vi "Configure Voltage.vi"(0 "VISA resource name":refnum<visa-resource-name>, 1 "DB Reference (1)":dbl=1.0, 2 "Input Impedance (0: 10Mohm)":i32(ring) items=["10Mohm", "Auto"], 5 "Function (0: Voltage DC)":i32(ring) items=["Voltage DC"=0, "Voltage AC"=1, "Digitize Voltage"=13], 9 "Channel List(\"\")":string, 11 "error in (no error)":errorcluster, 12 "Unit (0: Volt)":i32(ring) items=["Volt", "DB"]) -> (4 "VISA resource name out":refnum<visa-resource-name>, 15 "error out":errorcluster)   [LabVIEW 2024, in "Keithley DMM6500 DAQ6500 Series.lvlib"]
doc: "Configures voltage settings, including DB reference, input impedance and unit."
uses:
  Keithley DMM6500 DAQ6500 Series.lvlib
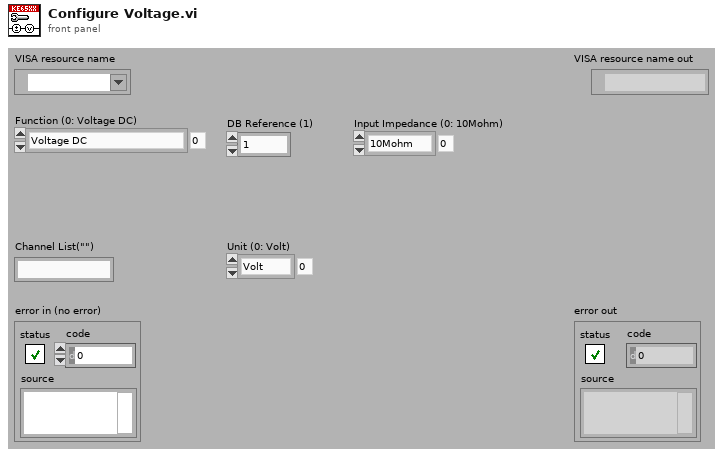
[diagram p1: front panel]
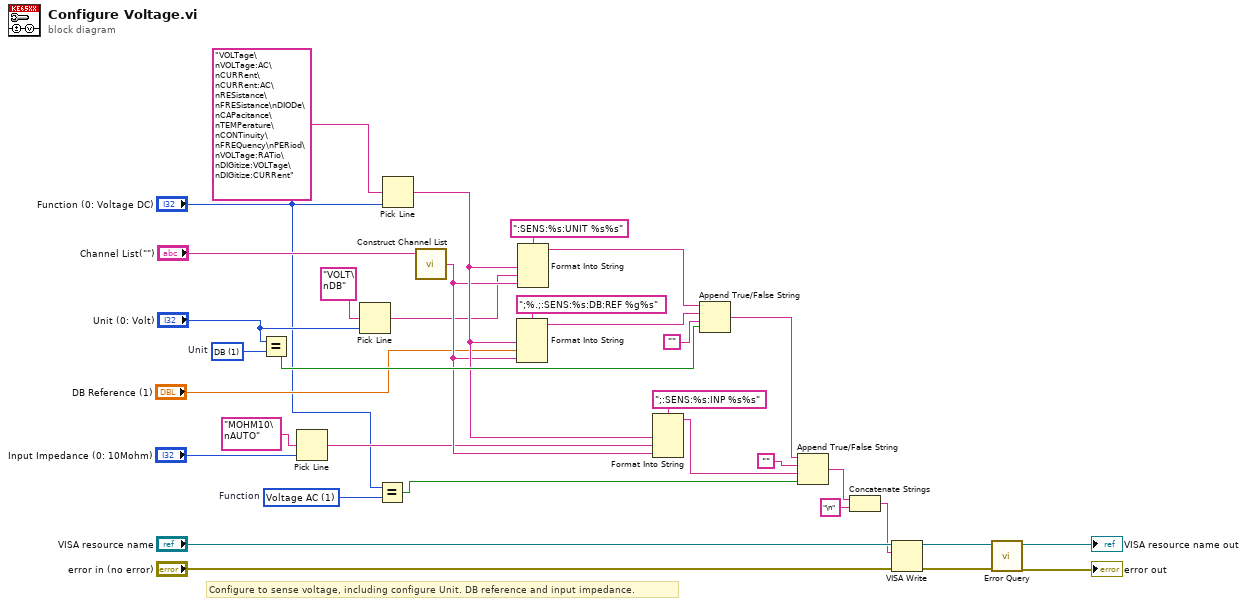
[diagram p0: block diagram]
diagram:
  w8 = u8 1 items=["Voltage DC"=0, "Voltage AC"=1, "Digitize Voltage"=13]  # Function
  w24 = u8 1 items=["VOLT", "DB"]  # Unit
  # "Configure to sense voltage, including configure Unit. DB reference and input impedance."
  n1 = Equal?(x="Unit (0: Volt)", y=w24) -> (x = y?=w22:bool)
  n2 = Pick Line(multi-line string="MOHM10\nAUTO", line index="Input Impedance (0: 10Mohm)") -> (output string=w10:string)  [unwired: 1 in]
  n3 = Pick Line(multi-line string="VOLT\nDB", line index="Unit (0: Volt)") -> (output string=w14:string)  [unwired: 1 in]
  n4 = Equal?(x="Function (0: Voltage DC)", y=w8) -> (x = y?=w7:bool)
  n5 = Pick Line(multi-line string="VOLTage\nVOLTage:AC\nCURRent\nCURRent:AC\nRESistance\nFRESistance\nDIODe\nCAPacitance\nTEMPerature\nCONTinuity\nFREQuency\nPERiod\nVOLTage:RATio\nDIGitize:VOLTage\nDIGitize:CURRent", line index="Function (0: Voltage DC)") -> (output string=w20:string)  [unwired: 1 in]
  n6 = call "Construct Channel List.vi"("Channel List"="Channel List(\"\")") -> ("Channel List String"=w19:string)  [unwired: 2 in]
  n7 = Format Into String(format string=";%.;:SENS:%s:DB:REF %g%s", w20, "DB Reference (1)", w19) -> (resulting string=w17:string)  [unwired: 2 in, 1 out]
  n8 = Format Into String(format string=":SENS:%s:UNIT %s%s", w20, w14, w19) -> (resulting string=w18:string)  [unwired: 2 in, 1 out]
  n9 = Format Into String(format string=";:SENS:%s:INP %s%s", w20, w10, w19) -> (resulting string=w6:string)  [unwired: 2 in, 1 out]
  n10 = Append True/False String(1:w22, 2:"" ("false string"), 3:w17, 4:w18) -> (0:w5:string)
  n11 = Append True/False String(1:w7, 2:w6, 3:"", 4:w5) -> (0:w2:string)
  n12 = Concatenate Strings(w2, "\n" ("string")) -> (w3:string)
  n13 = VISA Write(VISA resource name="VISA resource name", write buffer=w3, error in (no error)="error in (no error)") -> (VISA resource name out=w29:refnum<visa-resource-name>, error out=w28:errorcluster)  [unwired: 1 out]
  n14 = call "Error Query.vi"("error in (no error)"=w28, "VISA resource name"=w29) -> ("error out"=→"error out":errorcluster, "VISA resource name out"=→"VISA resource name out":refnum<visa-resource-name>)  [unwired: 6 in, 2 out]
